vi "Prompting.vi"(6 "menu reference":refnum<k9>, 7 "Command":T3=enum."INIT", 8 "error in (no error)":errorcluster, 10 "StartLotTraveler":T1, 11 "EpiWrapper in":refnum<class "EpiWrapper.lvclass">) -> (0 "error out":errorcluster, 3 "EpiWrapper out":refnum<class "EpiWrapper.lvclass">)   [LabVIEW 2012, in "EpiWrapper.lvclass"]
uses:
  EpiWrapper.lvclass
  Controls/Command_Enum.ctl
  LotData.lvclass
  Instruments.lvclass
  Controls/StartLotTraveler.ctl
  Controls/MeasurementType.ctl
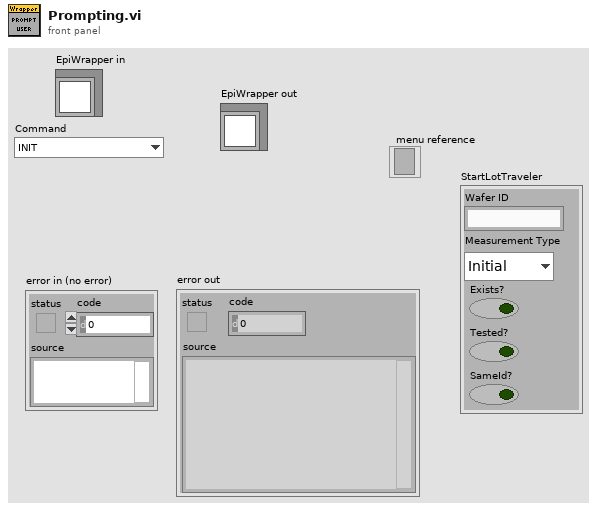
[diagram p1: front panel]
types:
  T1 = typedef "StartLotTraveler.ctl" = cluster{"Wafer ID":string, "Measurement Type":T2, "Exists?":bool, "Tested?":bool, "SameId?":bool}
  T2 = typedef "MeasurementType.ctl" = enum16{"Initial", "Final"}
  T3 = typedef "Command_Enum.ctl" = enum16{"SPECTRUMCAPTURE", "INSITUMEASURE", "RESETCONFIG", "OPENCONFIG", "RESET", "INIT", "LOAD", "MEASURE", "NEW", "SAVE", "UPDATE_INT", "SWAP_MODE", "UPDATE_ACQ", "MARK_MAP_SELECT", "MARK_MAP", "EXIT", "CANCEL"}
  T4 = enum8{"Enabled", "Disabled", "Disabled and Grayed Out"}
  T5 = typedef "CurrentPad.ctl" = cluster{"Coords":cluster{"Horizontal":sgl, "Vertical":sgl}, "radius":i32, "Tested":bool, "Selected":bool, "Pad":string, "PadArea":T6}
  T6 = typedef "PadArea.ctl" = enum16{"A", "B", "C", "D", "L", "R", "T", "G"}
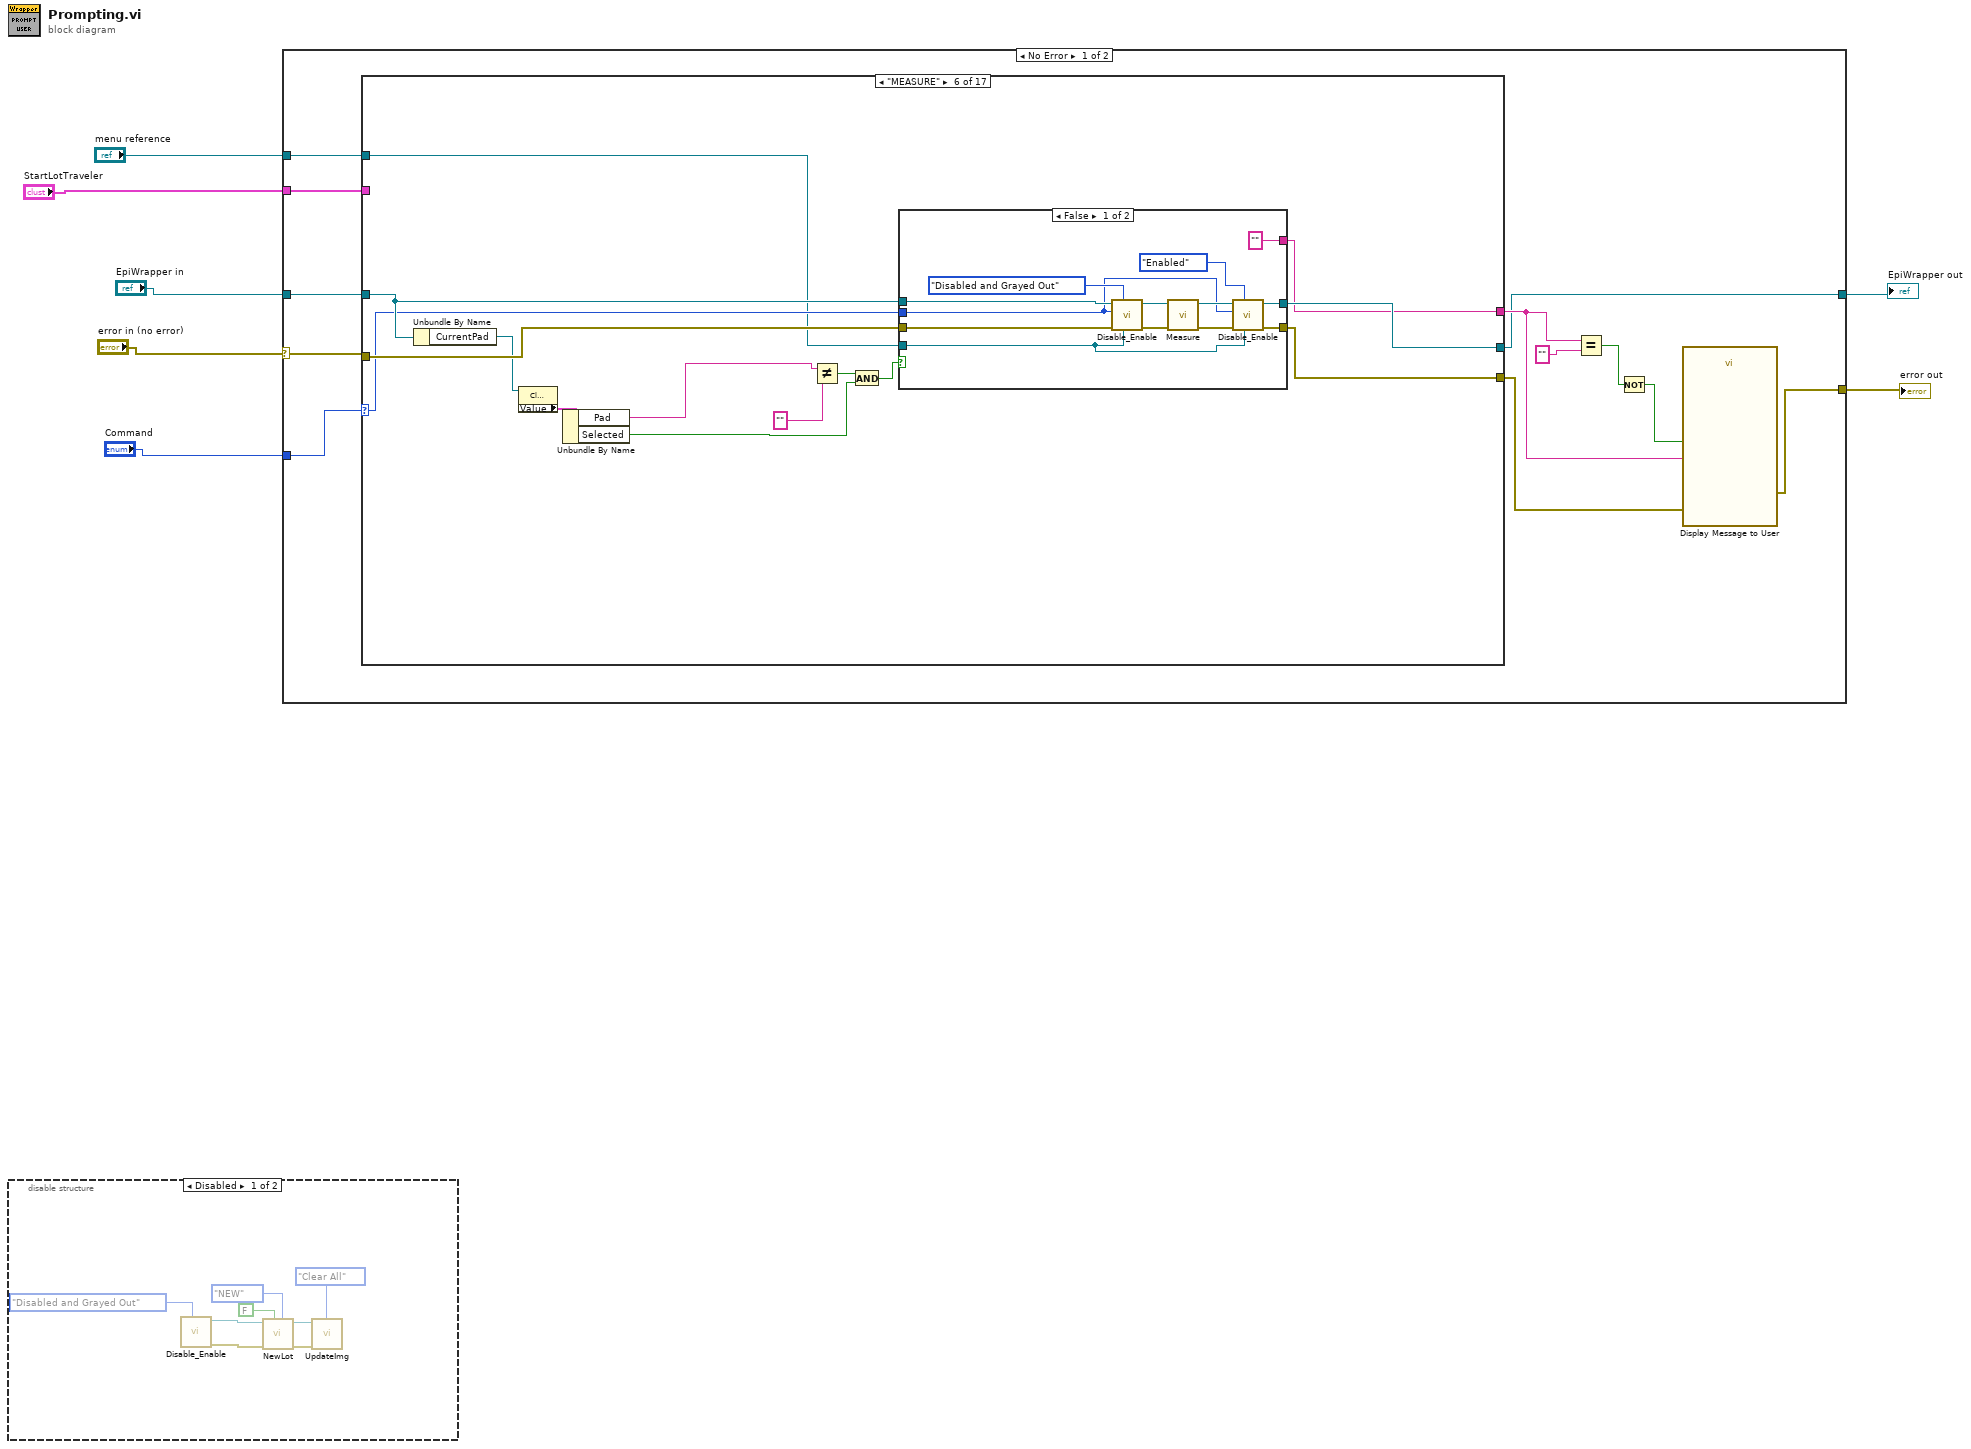
[diagram p0: block diagram]
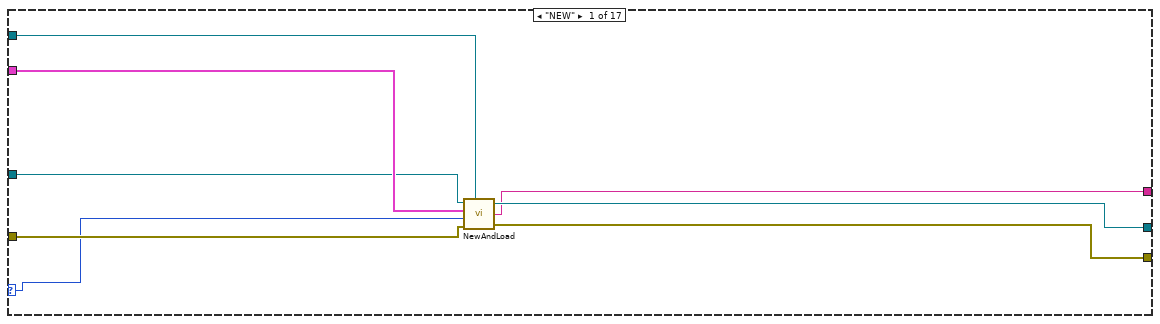
[diagram p3: hidden frame]
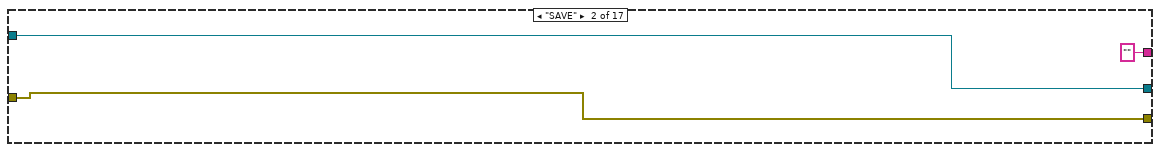
[diagram p4: hidden frame]
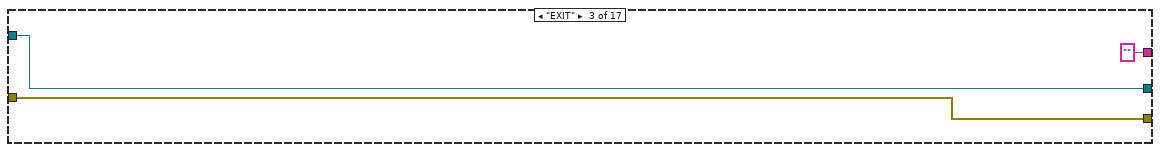
[diagram p5: hidden frame]
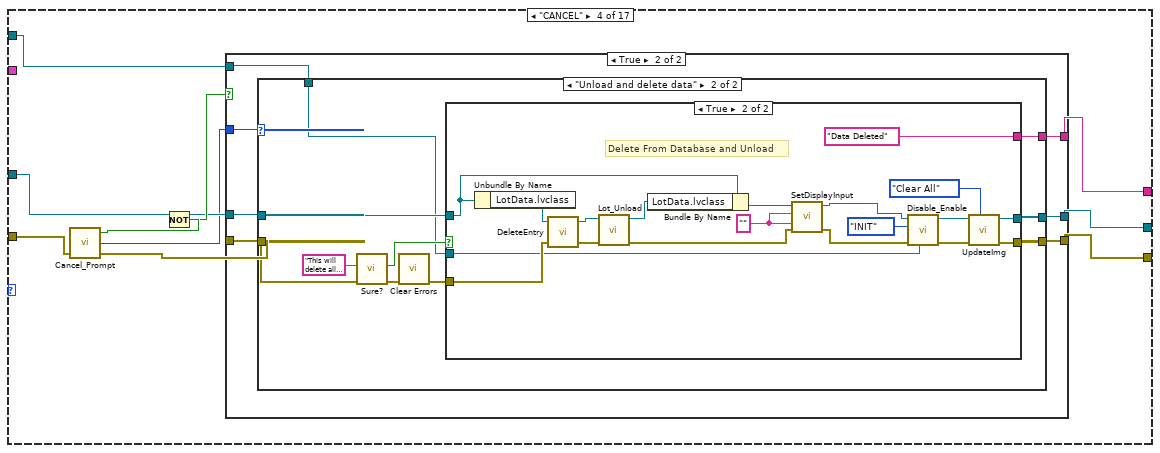
[diagram p6: hidden frame]
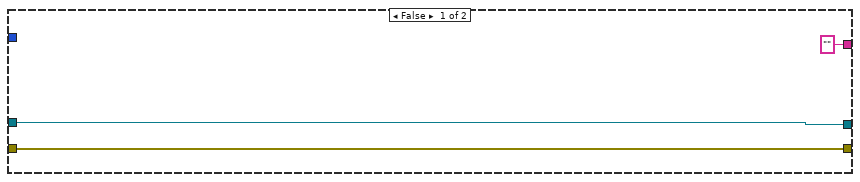
[diagram p7: hidden frame]
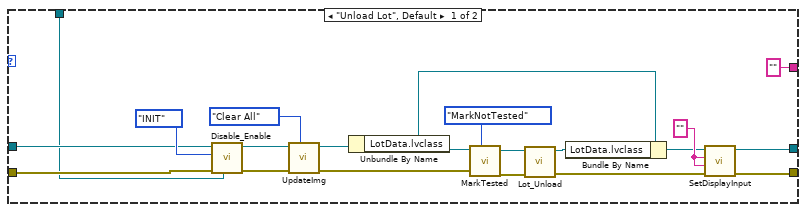
[diagram p8: hidden frame]
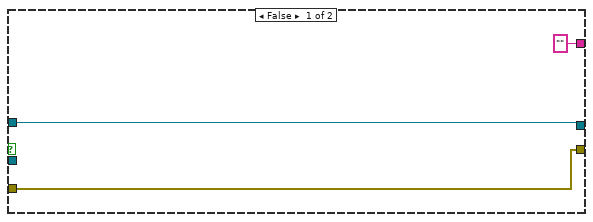
[diagram p9: hidden frame]
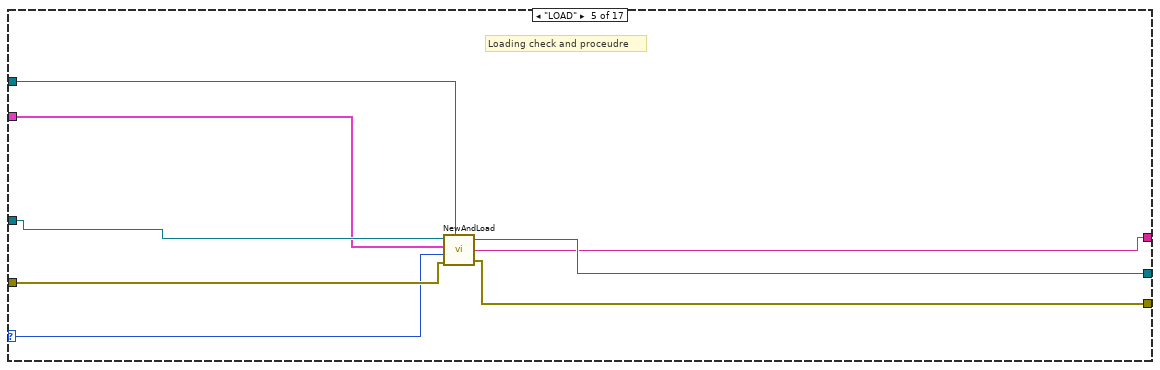
[diagram p10: hidden frame]
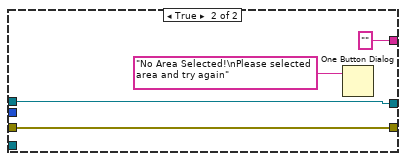
[diagram p11: hidden frame]
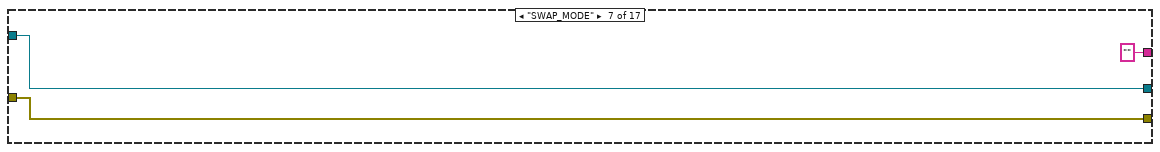
[diagram p12: hidden frame]
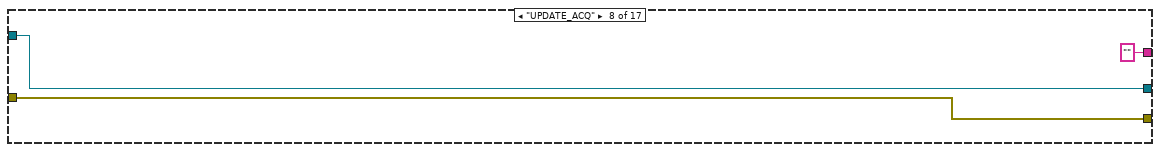
[diagram p13: hidden frame]
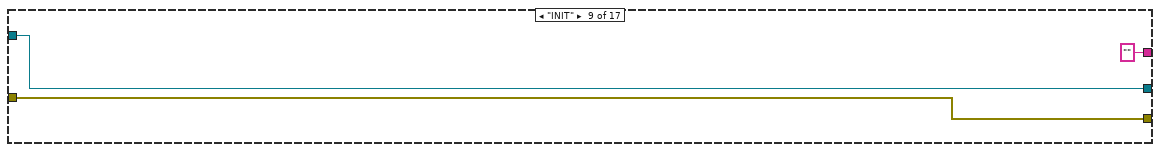
[diagram p14: hidden frame]
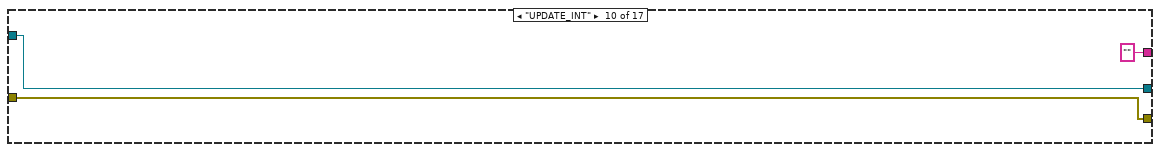
[diagram p15: hidden frame]
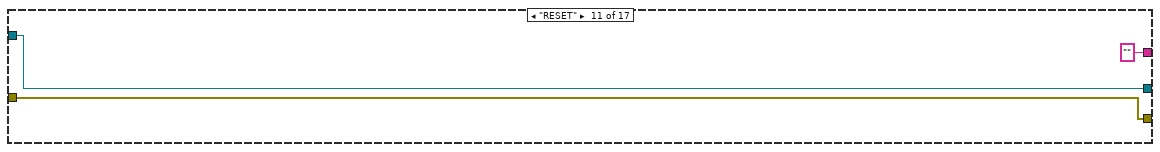
[diagram p16: hidden frame]
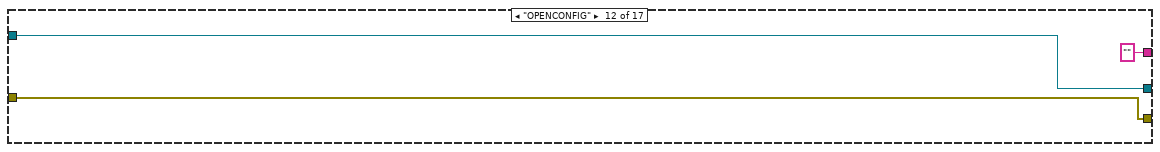
[diagram p17: hidden frame]
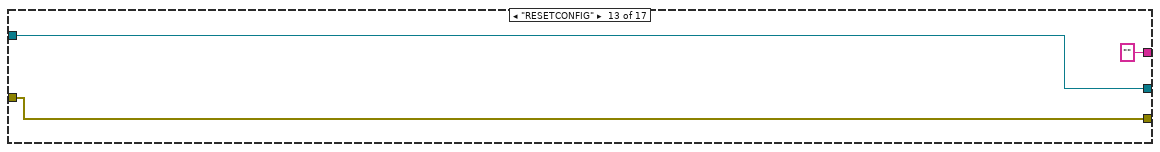
[diagram p18: hidden frame]
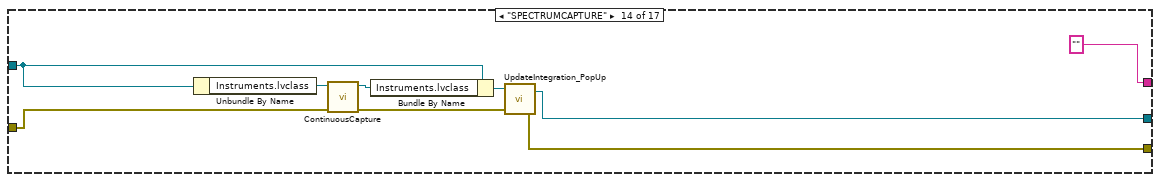
[diagram p19: hidden frame]
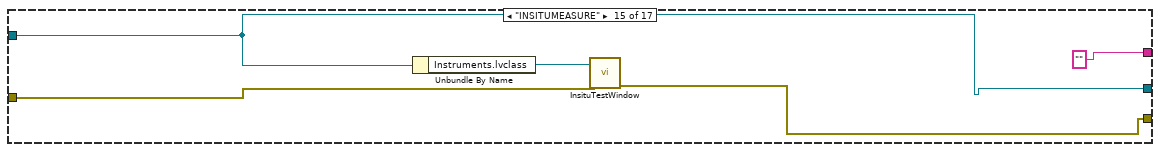
[diagram p20: hidden frame]
diagram:
  n1 = disable-structure shown="Disabled" {
    frame Disabled {
      n2 = call-dynamic "Disable_Enable.vi"("Disabled"=T4."Disabled and Grayed Out") -> ("error out"=w12:errorcluster, "EpiWrapper out"=w14:refnum<class "EpiWrapper.lvclass">)  [unwired: 9 in]
      n3 = call-dynamic "NewLot.vi"("Enum"=enum16{"LOAD", "NEW"}."NEW", "Create Entry?"=FALSE, "error in (no error)"=w12, "FrontPanelData in"=w14) -> ("error out"=w13:errorcluster, "FrontPanelData out"=w15:refnum<class "EpiWrapper.lvclass">)  [unwired: 5 in, 1 out]
      n4 = call-dynamic "UpdateImg.vi"("Enum"=enum16{"Mark", "Clear All"}."Clear All", "error in (no error)"=w13, "EpiWrapper in"=w15) -> ()  [unwired: 7 in, 2 out]
    }
    frame Enabled {
    }
  }
  n5 = case shown="No Error" "error in (no error)" {
    selector: "error in (no error)" -> [w25 w195]
    tunnel: [w19 w195] -> w6
    tunnel: [w18 w194] -> w4
    tunnel: "EpiWrapper in" -> [w26 w194]
    tunnel: "Command" -> [w27 _]
    tunnel: "menu reference" -> [w17 _]
    tunnel: "StartLotTraveler" -> [w16 _]
    frame No Error {
      n6 = case shown="\"MEASURE\"" w27 {
        selector: w27 -> [w32 _ _ _ w118 w131 _ _ _ _ _ _ _ _ _ _ _]
        tunnel: [w30 w37 w40 w47 w117 w133 w154 w157 w160 w163 w165 w168 w172 w176 w184 w188 w192] -> w20
        tunnel: w26 -> [w34 w38 w41 w48 w121 w135 w155 w158 w161 w164 w166 w170 w173 w180 w185 w190 w193]
        tunnel: w25 -> [w33 w37 w40 w51 w119 w134 w154 w157 w160 w163 w165 w168 w172 w181 w186 w188 w192]
        tunnel: [w31 w38 w41 w45 w116 w132 w155 w158 w161 w164 w166 w170 w173 w175 w185 w190 w193] -> w18
        tunnel: [w29 "" "" w43 w115 w130 "" "" "" "" "" "" "" "" "" "" "" ("Message")] -> w23
        tunnel: w17 -> [w28 _ _ w42 w114 w129 _ _ _ _ _ _ _ _ _ _ _]
        tunnel: w16 -> [w35 _ _ _ w120 _ _ _ _ _ _ _ _ _ _ _ _]
        frame "NEW" {
          n7 = call-dynamic "NewAndLoad.vi"("EpiWrapper in"=w34, "StartLotTraveler"=w35, "Command"=w32, "error in (no error)"=w33, "menu reference"=w28) -> ("EpiWrapper out"=w31:refnum<class "EpiWrapper.lvclass">, "Message"=w29:string, "error out"=w30:errorcluster)
        }
        frame "SAVE" {
        }
        frame "EXIT" {
        }
        frame "CANCEL" {
          n8 = call "Cancel_Prompt.vi"("error in (no error)"=w51) -> ("error out"=w46:errorcluster, "Enum 2"=w44:enum16{"Unload Lot", "Unload and delete data"}, "Cancelled?"=w50:bool)  [unwired: 2 in]
          n9 = Not(x=w50) -> (.not. x?=w49:bool)
          n10 = case shown="True" w49 {
            tunnel: w44 -> [_ w61]
            tunnel: w48 -> [w54 w60]
            tunnel: [w53 w58] -> w47
            tunnel: w46 -> [w53 w59]
            tunnel: [w54 w57] -> w45
            tunnel: ["" w56] -> w43
            tunnel: w42 -> [_ w55]
            frame False {
            }
            frame True {
              n11 = case shown="\"Unload and delete data\"" w61 {
                tunnel: w60 -> [w78 w91]
                tunnel: w59 -> [w77 w86]
                tunnel: [w67 w90] -> w58
                tunnel: [w68 w89] -> w57
                tunnel: ["" w83] -> w56
                tunnel: w55 -> [w63 w82]
                frame "Unload Lot", Default {
                  w69 = "" ("Wafer ID")
                  n12 = call-dynamic "Disable_Enable.vi"("menu reference"=w63, "error in (no error)"=w77, "Command"=Command_Enum."INIT", "EpiWrapper in"=w78) -> ("error out"=w79:errorcluster, "EpiWrapper out"=w80:refnum<class "EpiWrapper.lvclass">)  [unwired: 6 in]
                  n13 = call-dynamic "UpdateImg.vi"("Enum"=enum16{"Remove", "Mark", "Clear All"}."Clear All", "error in (no error)"=w79, "EpiWrapper in"=w80) -> ("error out"=w70:errorcluster, "EpiWrapper out"=w71:refnum<class "EpiWrapper.lvclass">)  [unwired: 7 in]
                  n14 = Unbundle By Name(w71) -> ("LotData.lvclass"=w72:refnum<class "LotData.lvclass">)
                  n15 = call-dynamic "MarkTested.vi"("Enum"=enum16{"MarkTested", "MarkNotTested"}."MarkNotTested", "error in (no error)"=w70, "LotData in"=w72) -> ("error out"=w74:errorcluster, "LotData out"=w75:refnum<class "LotData.lvclass">)  [unwired: 6 in, 1 out]
                  n16 = call-dynamic "Lot_Unload.vi"("error in (no error)"=w74, "LotData in"=w75) -> ("error out"=w65:errorcluster, "LotData out"=w76:refnum<class "LotData.lvclass">)  [unwired: 8 in]
                  n17 = Bundle By Name(cluster=w71, "LotData.lvclass"=w76) -> (w66:refnum<class "EpiWrapper.lvclass">)
                  n18 = call-dynamic "SetDisplayInput.vi"("error in (no error)"=w65, "Test"=w69, "Wafer ID"=w69, "EpiWrapper in"=w66) -> ("error out"=w67:errorcluster, "EpiWrapper out"=w68:refnum<class "EpiWrapper.lvclass">)  [unwired: 6 in]
                }
                frame "Unload and delete data" {
                  n19 = call "Sure?"("error in (no error)"=w86, "Message"="This will delete all data associated with this wafer.\n\nAre you absolutly sure you want to continue?") -> ("error out"=w87:errorcluster, "YES,DELETE DATA"=w85:bool)  [unwired: 8 in]
                  n20 = call <vilib>:"Clear Errors.vi"("error in (no error)"=w87) -> ("error out"=w84:errorcluster)  [unwired: 6 in]
                  n21 = case shown="True" w85 {
                    tunnel: w91 -> [w94 w107]
                    tunnel: [w93 w105] -> w90
                    tunnel: [w94 w104] -> w89
                    tunnel: w84 -> [w93 w98]
                    tunnel: ["" "Data Deleted"] -> w83
                    tunnel: w82 -> [_ w96]
                    frame False {
                    }
                    frame True {
                      w102 = "" ("Wafer ID")
                      # "Delete From Database and Unload"
                      n22 = Unbundle By Name(w107) -> ("LotData.lvclass"=w110:refnum<class "LotData.lvclass">)
                      n23 = call-dynamic "DeleteEntry.vi"("error in (no error)"=w98, "LotData in"=w110) -> ("error out"=w108:errorcluster, "LotData out"=w109:refnum<class "LotData.lvclass">)  [unwired: 1 in, 1 out]
                      n24 = call-dynamic "Lot_Unload.vi"("error in (no error)"=w108, "LotData in"=w109) -> ("error out"=w101:errorcluster, "LotData out"=w106:refnum<class "LotData.lvclass">)  [unwired: 8 in]
                      n25 = Bundle By Name(cluster=w107, "LotData.lvclass"=w106) -> (w103:refnum<class "EpiWrapper.lvclass">)
                      n26 = call-dynamic "SetDisplayInput.vi"("error in (no error)"=w101, "Test"=w102, "Wafer ID"=w102, "EpiWrapper in"=w103) -> ("error out"=w100:errorcluster, "EpiWrapper out"=w99:refnum<class "EpiWrapper.lvclass">)  [unwired: 6 in]
                      n27 = call-dynamic "Disable_Enable.vi"("menu reference"=w96, "error in (no error)"=w100, "Command"=Command_Enum."INIT", "EpiWrapper in"=w99) -> ("error out"=w111:errorcluster, "EpiWrapper out"=w112:refnum<class "EpiWrapper.lvclass">)  [unwired: 6 in]
                      n28 = call-dynamic "UpdateImg.vi"("Enum"=enum16{"Remove", "Mark", "Clear All"}."Clear All", "error in (no error)"=w111, "EpiWrapper in"=w112) -> ("error out"=w105:errorcluster, "EpiWrapper out"=w104:refnum<class "EpiWrapper.lvclass">)  [unwired: 7 in]
                    }
                  }
                }
              }
            }
          }
        }
        frame "LOAD" {
          # "Loading check and proceudre"
          n29 = call-dynamic "NewAndLoad.vi"("EpiWrapper in"=w121, "StartLotTraveler"=w120, "Command"=w118, "error in (no error)"=w119, "menu reference"=w114) -> ("EpiWrapper out"=w116:refnum<class "EpiWrapper.lvclass">, "Message"=w115:string, "error out"=w117:errorcluster)
        }
        frame "MEASURE" {
          n30 = Unbundle By Name(w135) -> ("CurrentPad"=w127:refnum<vi>)
          n31 = property class="Clust (strict)"(reference=w127) -> ("Value"=w126:T5)  [unwired: 1 in, 2 out]
          n32 = Unbundle By Name(w126) -> ("Pad"=w125:string, "Selected"=w122:bool)
          n33 = Not Equal?(x=w125, y="" ("Pad")) -> (x != y?=w124:bool)
          n34 = And(x=w124, y=w122) -> (x .and. y?=w123:bool)
          n35 = case shown="False" w123 {
            tunnel: w135 -> [w144 w151]
            tunnel: w134 -> [w143 w150]
            tunnel: [w142 w150] -> w133
            tunnel: [w141 w151] -> w132
            tunnel: w131 -> [w139 _]
            tunnel: ["" ""] -> w130
            tunnel: w129 -> [w136 _]
            frame False {
              n36 = call-dynamic "Disable_Enable.vi"("menu reference"=w136, "Disabled"=T4."Disabled and Grayed Out", "error in (no error)"=w143, "Command"=w139, "EpiWrapper in"=w144) -> ("error out"=w145:errorcluster, "EpiWrapper out"=w146:refnum<class "EpiWrapper.lvclass">)  [unwired: 5 in]
              n37 = call-dynamic "Measure.vi"("error in (no error)"=w145, "EpiWrapper in"=w146) -> ("error out"=w138:errorcluster, "EpiWrapper out"=w140:refnum<class "EpiWrapper.lvclass">)  [unwired: 8 in]
              n38 = call-dynamic "Disable_Enable.vi"("menu reference"=w136, "Disabled"=T4."Enabled", "error in (no error)"=w138, "Command"=w139, "EpiWrapper in"=w140) -> ("error out"=w142:errorcluster, "EpiWrapper out"=w141:refnum<class "EpiWrapper.lvclass">)  [unwired: 5 in]
            }
            frame True {
              n39 = One Button Dialog(message="No Area Selected!\nPlease selected area and try again") -> ()  [unwired: 1 in, 1 out]
            }
          }
        }
        frame "SWAP_MODE" {
        }
        frame "UPDATE_ACQ" {
        }
        frame "INIT" {
        }
        frame "UPDATE_INT" {
        }
        frame "RESET" {
        }
        frame "OPENCONFIG" {
        }
        frame "RESETCONFIG" {
        }
        frame "SPECTRUMCAPTURE" {
          n40 = Unbundle By Name(w180) -> ("Instruments.lvclass"=w182:refnum<class "Instruments.lvclass">)
          n41 = call-dynamic "ContinuousCapture.vi"("error in (no error)"=w181, "Instruments in"=w182) -> ("error out"=w174:errorcluster, "Instruments out"=w179:refnum<class "Instruments.lvclass">)  [unwired: 8 in]
          n42 = Bundle By Name(cluster=w180, "Instruments.lvclass"=w179) -> (w177:refnum<class "EpiWrapper.lvclass">)
          n43 = call-dynamic "UpdateIntegration_PopUp.vi"("error in (no error)"=w174, "EpiWrapper in"=w177) -> ("error out"=w176:errorcluster, "EpiWrapper out"=w175:refnum<class "EpiWrapper.lvclass">)  [unwired: 1 in]
        }
        frame "INSITUMEASURE" {
          n44 = Unbundle By Name(w185) -> ("Instruments.lvclass"=w187:refnum<class "Instruments.lvclass">)
          n45 = call-dynamic "InsituTestWindow.vi"("error in (no error)"=w186, "Instruments in"=w187) -> ("error out"=w184:errorcluster)  [unwired: 8 in, 1 out]
        }
        frame "MARK_MAP" {
        }
        frame "MARK_MAP_SELECT" {
        }
      }
      n46 = Equal?(x=w23, y="") -> (x = y?=w22:bool)
      n47 = Not(x=w22) -> (.not. x?=w21:bool)
      n48 = call "Display Message to User"("error in (no error)"=w20, "Enable"=w21, "Message"=w23) -> ("error out"=w19:errorcluster)  [unwired: 7 in, 1 out]
    }
    frame Error {
    }
  }
  "error out" <- w6
  "EpiWrapper out" <- w4
